vi "test_CCDSetAndGetNumberOfAverages.vi"   [LabVIEW 2023]
uses:
  <vilib>/addons/_JKI Toolkits/Caraya/classes/Test/Test.lvclass
  <vilib>/addons/_JKI Toolkits/Caraya/classes/Assert/Assert.lvclass
  Classes/CCD/CCD.lvclass
  Classes/CCD/NumberOfAverages.ctl
  <vilib>/addons/_JKI Toolkits/Caraya/classes/Assert/Assert Equal Value and Type_Variant.vi
  <vilib>/addons/_JKI Toolkits/Caraya/classes/Assert/Assert Not Error.vi
  <vilib>/addons/_JKI Toolkits/Caraya/classes/Assert/Assert Error.vi
types:
  T1 = typedef "CCD.lvclass/NumberOfAverages.ctl" = cluster{"number of averages":u32}
  T2 = typedef "CCD.lvclass/NumberOfAverages.ctl" = cluster{"number of averages":i32}
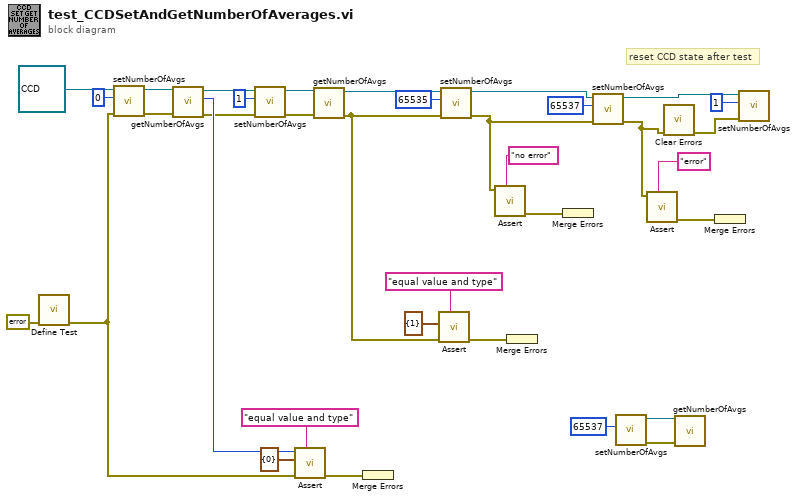
[diagram p0: block diagram]
diagram:
  # "reset CCD state after test"
  n1 = call <vilib>:"Define Test.vi"("error in (no error)"=errorcluster {"status"=FALSE, "code"=0, "source"=""}) -> ("error out"=w28:errorcluster)  [unwired: 9 in, 1 out]
  n2 = call "setNumberOfAvgs.vi"("error in (no error)"=w28, "number of averages"=0, "CCD in"=refnum<class "CCD.lvclass"> refnum) -> ("error out"=w27:errorcluster, "CCD out"=w29:refnum<class "CCD.lvclass">)  [unwired: 5 in, 2 out]
  n3 = call "getNumberOfAvgs.vi"("error in (no error)"=w27, "CCD in"=w29) -> ("error out"=w14:errorcluster, "number of averages"=w32:i32, "CCD out"=w18:refnum<class "CCD.lvclass">)  [unwired: 7 in]
  n4 = call "setNumberOfAvgs.vi"("error in (no error)"=w14, "number of averages"=1, "CCD in"=w18) -> ("error out"=w24:errorcluster, "CCD out"=w25:refnum<class "CCD.lvclass">)  [unwired: 5 in, 2 out]
  n5 = call-poly <vilib>:"Assert.vi"("Label"="equal value and type" ("Label (VI Title)"), "error in (no error)"=w28, "Y"=T2 {"number of averages"=0} ("Averaging"), "X"=w32) -> ("error out"=w34:errorcluster)  [unwired: 6 in, 1 out]
  n6 = call "getNumberOfAvgs.vi"("error in (no error)"=w24, "CCD in"=w25) -> ("error out"=w10:errorcluster, "CCD out"=w13:refnum<class "CCD.lvclass">)  [unwired: 7 in, 1 out]
  n7 = Merge Errors(w34) -> ()  [unwired: 1 out]
  n8 = call-poly <vilib>:"Assert.vi"("Label"="equal value and type" ("Label (VI Title)"), "error in (no error)"=w10, "Y"=T1 {"number of averages"=1} ("Averaging")) -> ("error out"=w16:errorcluster)  [unwired: 7 in, 1 out]
  n9 = call "setNumberOfAvgs.vi"("error in (no error)"=w10, "number of averages"=65535, "CCD in"=w13) -> ("error out"=w3:errorcluster, "CCD out"=w6:refnum<class "CCD.lvclass">)  [unwired: 5 in, 2 out]
  n10 = call-poly <vilib>:"Assert.vi"("Label"="no error" ("Label (VI Title)"), "Not Error?"=w3) -> ("error out"=w11:errorcluster)  [unwired: 8 in, 1 out]
  n11 = Merge Errors(w16) -> ()  [unwired: 1 out]
  n12 = Merge Errors(w11) -> ()  [unwired: 1 out]
  n13 = call "setNumberOfAvgs.vi"("error in (no error)"=w3, "number of averages"=65537, "CCD in"=w6) -> ("error out"=w2:errorcluster, "CCD out"=w4:refnum<class "CCD.lvclass">)  [unwired: 5 in, 2 out]
  n14 = call "setNumberOfAvgs.vi"("number of averages"=65537) -> ("error out"=w20:errorcluster, "CCD out"=w21:refnum<class "CCD.lvclass">)  [unwired: 7 in, 2 out]
  n15 = call-poly <vilib>:"Assert.vi"("Label"="error" ("Label (VI Title)"), "Error?"=w2) -> ("error out"=w7:errorcluster)  [unwired: 8 in, 1 out]
  n16 = call <vilib>:"Clear Errors.vi"("error in (no error)"=w2) -> ("error out"=w1:errorcluster)  [unwired: 5 in, 1 out]
  n17 = call "getNumberOfAvgs.vi"("error in (no error)"=w20, "CCD in"=w21) -> ()  [unwired: 7 in, 3 out]
  n18 = Merge Errors(w7) -> ()  [unwired: 1 out]
  n19 = call "setNumberOfAvgs.vi"("error in (no error)"=w1, "number of averages"=1, "CCD in"=w4) -> ()  [unwired: 5 in, 4 out]
